vi "Easy Print VI Panel or Documentation.vi"   [LabVIEW 2017, in "NI_ReportGenerationCore.lvlib"]
doc: "Prints a front panel or VI documentation or saves the front panel or VI documentation to a report. Wire data to the <B>VI path</B> input to determine the polymorphic instance to use or manually select the instance."
uses:
  <vilib>/Utility/NIReport.llb/NI_ReportGenerationCore.lvlib
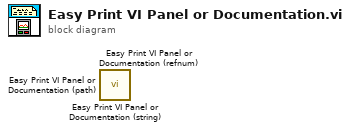
[diagram p0: block diagram]
diagram:
  n1 = call <vilib>:"Easy Print VI Panel or Documentation (string).vi"() -> ()  [unwired: 10 in, 2 out]
  n2 = call <vilib>:"Easy Print VI Panel or Documentation (refnum).vi"() -> ()  [unwired: 10 in, 2 out]
  n3 = call <vilib>:"Easy Print VI Panel or Documentation (path).vi"() -> ()  [unwired: 10 in, 2 out]
